vi "doAction.vi"(8 "error in (no error)":errorcluster, 10 "ContextData":refnum<class "ContextData.lvclass">, 11 "Run in":refnum<class "Play Game.lvclass">) -> (0 "error out":errorcluster, 2 "ContextData Out":refnum<class "ContextData.lvclass">, 3 "Run out":refnum<class "Play Game.lvclass">)   [LabVIEW 2019, in "Play Game.lvclass"]
uses:
  Play Game.lvclass
  ContextData/ContextData.lvclass
  Simon_Engine/Simon_Engine.lvclass
  Messages/simonMessages/simonMessages.lvclass
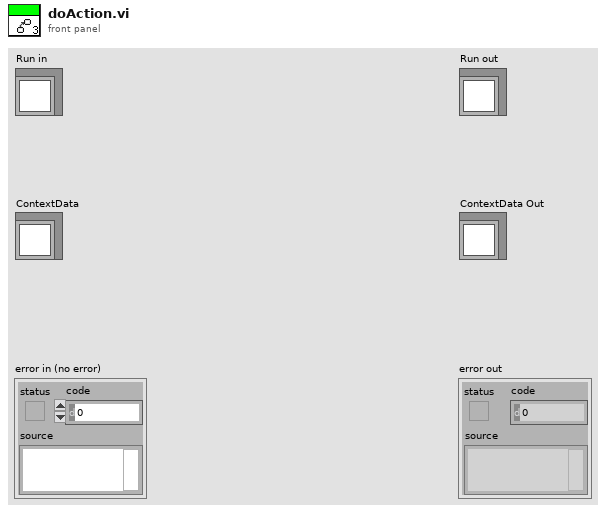
[diagram p1: front panel]
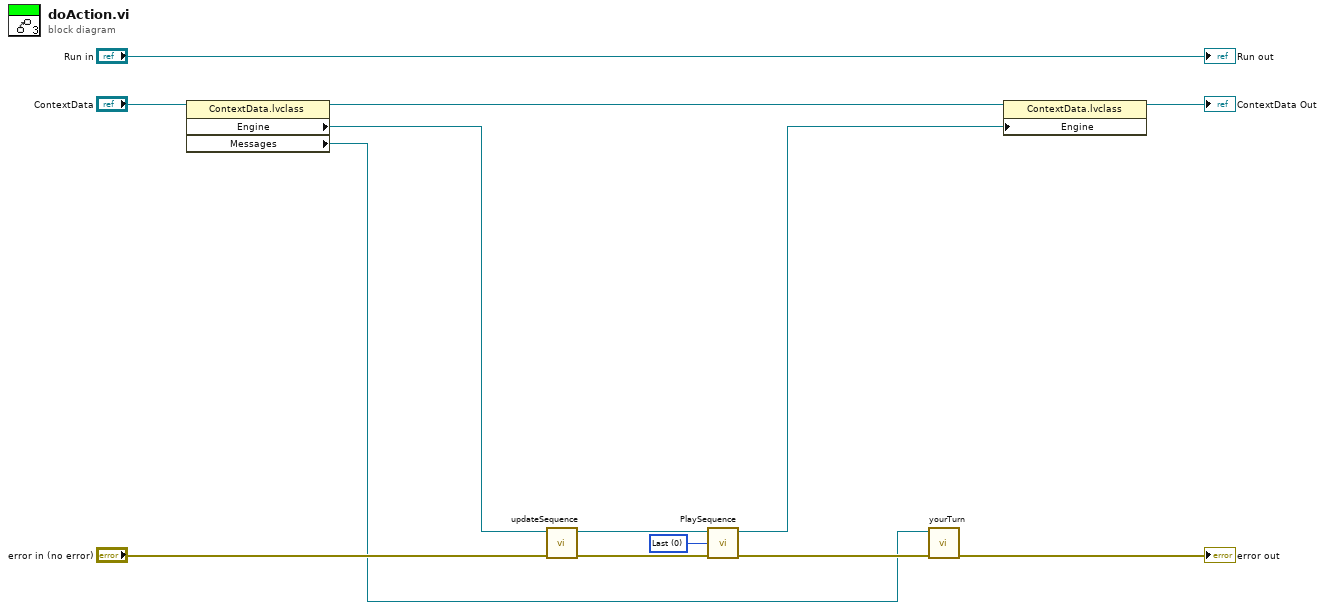
[diagram p0: block diagram]
diagram:
  w9 = u8 0 items=["Last", "Longest"] ("Sequence")
  n1 = property class="ContextData.lvclass"(reference="ContextData") -> (reference out=w11:refnum<class "ContextData.lvclass">, "Engine"=w2:refnum<class "Simon_Engine.lvclass">, "Messages"=w1:refnum<class "simonMessages.lvclass">)  [unwired: 1 in, 1 out]
  n2 = call-dynamic "updateSequence.vi"("error in (no error)"="error in (no error)", "Simon_Engine in"=w2) -> ("error out"=w6:errorcluster, "Simon_Engine out"=w5:refnum<class "Simon_Engine.lvclass">)  [unwired: 8 in]
  n3 = call-dynamic "PlaySequence.vi"("error in (no error)"=w6, "Sequence"=w9, "Simon_Engine in"=w5) -> ("error out"=w8:errorcluster, "Simon_Engine out"=w7:refnum<class "Simon_Engine.lvclass">)  [unwired: 7 in]
  n4 = call "yourTurn.vi"("error in (no error)"=w8, "simonMessages in"=w1) -> ("error out"=→"error out":errorcluster)  [unwired: 8 in, 1 out]
  n5 = property class="ContextData.lvclass"(reference=w11, "Engine"=w7) -> (reference out=→"ContextData Out":refnum<class "ContextData.lvclass">)  [unwired: 1 in, 1 out]
  "Run out" <- "Run in"
